vi "S7_Init_TCP.vi"(8 "error in":errorcluster, 9 "Connection Timeout":u32=5000, 11 "IP Address":string) -> (0 "error out":errorcluster, 3 "TCP Connection Ref":refnum<k5>)   [LabVIEW 2017, in "S7 TCP.lvlib"]
uses:
  S7 TCP.lvlib
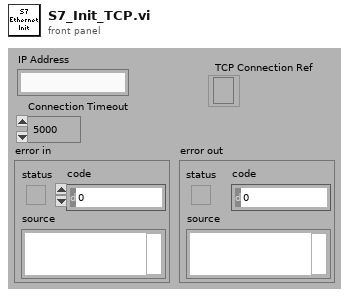
[diagram p1: front panel]
types:
  T1 = enum16{"Standard", "Buffered", "CRLF", "Immediate"}
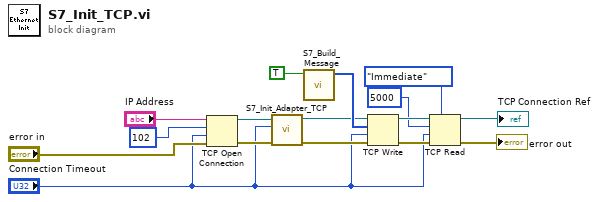
[diagram p0: block diagram]
diagram:
  n1 = TCP Open Connection(address="IP Address", remote port or service name=u16 102, timeout ms (60000)="Connection Timeout", error in (no error)="error in") -> (connection ID=w13:refnum<k5>, error out=w12:errorcluster)  [unwired: 1 out]
  n2 = call "S7_Init_Adapter_TCP.vi"("error in"=w12, "Timeout"="Connection Timeout", "TCP Connection Ref"=w13) -> ("error out"=w10:errorcluster, "TCP Connection Ref Out"=w9:refnum<k5>)  [unwired: 7 out]
  n3 = call "S7_Build_Message.vi"("Exchange PDU"=TRUE) -> ("S7 Ethernet Data"=w11:u8[])  [unwired: 2 in, 8 out]
  n4 = TCP Write(connection ID=w9, data in=w11, error in (no error)=w10, 9:"Connection Timeout") -> (connection ID out=w7:refnum<k5>, error out=w6:errorcluster)  [unwired: 1 out]
  n5 = TCP Read(connection ID=w7, bytes to read=5000, error in (no error)=w6, 7:T1."Immediate" ("mode (standard)"), 9:"Connection Timeout") -> (connection ID out=→"TCP Connection Ref":refnum<k5>, error out=→"error out":errorcluster)  [unwired: 1 out]
